vi "swmm_step.vi"(3 "error in (no error)":errorcluster) -> (0 "error out":errorcluster, 2 "new_elapsed_time":dbl)   [LabVIEW 2014]
uses:
  swmm5.dll
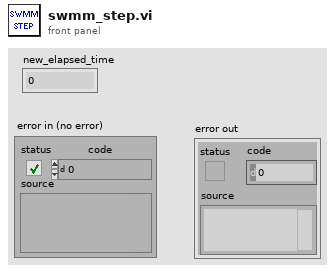
[diagram p1: front panel]
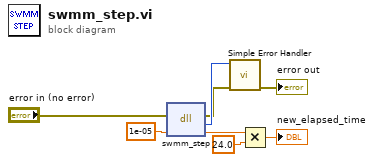
[diagram p0: block diagram]
diagram:
  n1 = dll-call lib="PTH2zabs CUsers\nandres riañoDropboxProyecto AguasSoftwareMatSWMMMatSWMM 5.1.009LabVIEW modulex64\tswmm5.dll" fn="swmm_step"(error in="error in (no error)", "elapsed_time"=1e-05) -> (error out=w1:errorcluster, "return type"=w8:i32, "elapsed_time"=w6:dbl)  [unwired: 2 in, 1 out]
  n2 = call <vilib>:"Simple Error Handler.vi"("error code (no error:0)"=w8, "error in (no error)"=w1) -> ("error out"=→"error out":errorcluster)  [unwired: 3 in, 4 out]
  n3 = Multiply(x=w6, y=24.0) -> (x*y=→"new_elapsed_time":dbl)
